vi "GetNumberOfRecords.vi"(8 "error in (no error)":errorcluster, 11 "FpgaRef5782 in":refnum<class "FpgaRefx410.lvclass">) -> (0 "error out":errorcluster, 2 "number of records":i32, 3 "FpgaRef5782 out":refnum<class "FpgaRefx410.lvclass">)   [LabVIEW 2025, in "FpgaRefx410.lvclass"]
uses:
  FpgaRefx410.lvclass
  FpgaRefx410.lvclass/FpgaRefx410.ctl
  <vilib>/Utility/error.llb/Error Cluster From Error Code.vi
  <vilib>/rvi/errors/niLvFpgaAdjustHostInterfaceError.vi
  <vilib>/rvi/interface/nirviMethod/nirviMethod.xnode
  x410 FPGA ref.ctl
  <vilib>/FPGAPlugInAG/Dynamic/niLvFpga_ReadFifo_Dynamic.vi
  <vilib>/rvi/errors/niLvFpgaMergeErrorWithErrorCode.vi
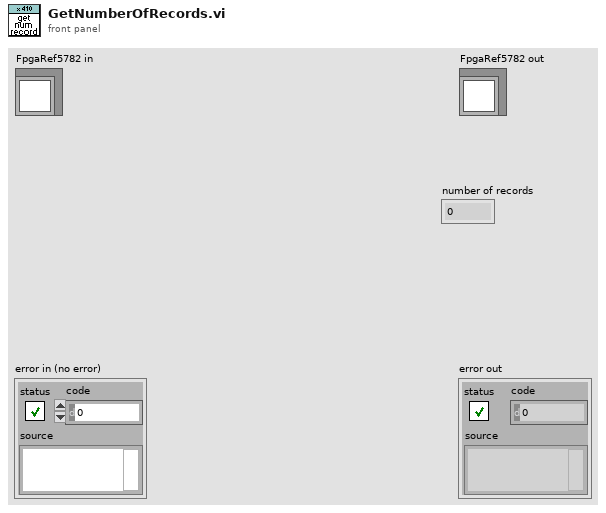
[diagram p1: front panel]
types:
  T1 = typedef "x410 FPGA ref.ctl" = refnum<k20>
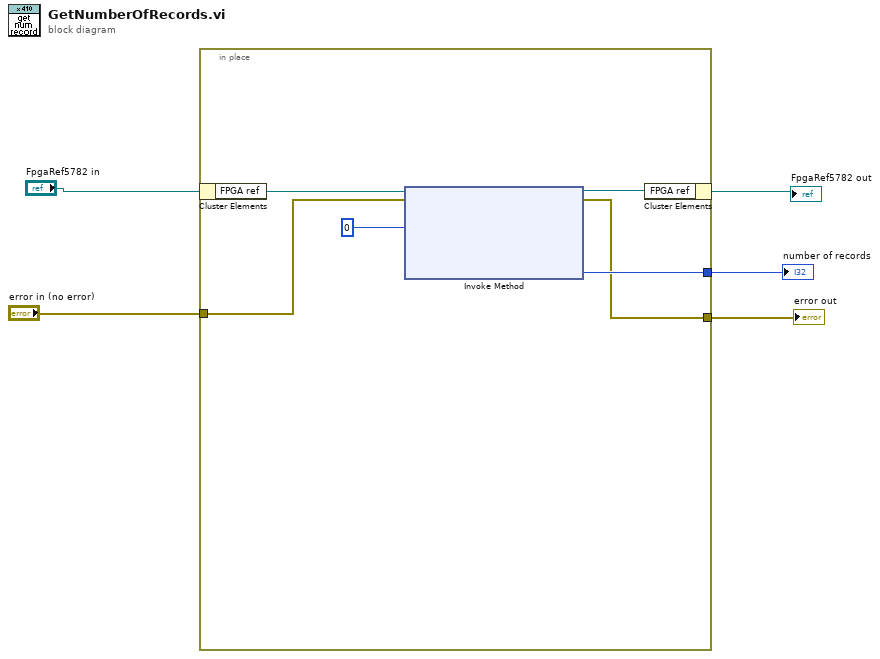
[diagram p0: block diagram]
diagram:
  n1 = in-place {
    in-place-border: [w8] -> w4
    in-place-border: "error in (no error)" -> [w7]
    in-place-border: [w6] -> w1
    n2 = in-place-cluster #1("FpgaRef5782 in") -> ("FPGA ref"=w10:T1)
    n3 = xnode "Invoke Method"("FPGA VI Reference In"=w10, "error in"=w7, "Number of Elements"=u32 0) -> ("FPGA VI Reference Out"=w9:T1, "error out"=w6:errorcluster, "Elements Remaining"=w8:u32)  [unwired: 1 in, 1 out]
    n4 = in-place-cluster #1("FPGA ref"=w9) -> (→"FpgaRef5782 out":refnum<class "FpgaRefx410.lvclass">)
  }
  "error out" <- w1
  "number of records" <- w4
